vi "Weather Station UI_EX.vi"() -> ()   [LabVIEW 2021]
doc: "This is the main VI in the Weather Station project. It contains the user interface for a temperature warning system. Temperature is retrieved every half second; data is logged when a warning has occurred."
uses:
  WeatherData.ctl
  Instance           2 26Saved   Weather Station UI .vi
panel:
  out "Warning":string
  in  "Lower Limit":dbl=20.0
  in  "Upper Limit":dbl=30.0
  in  "Stop Button":bool
  out "Temperature History":dbl(graph)
  # "Temperature Ranges (C)"
  # "Freeze"
  # "Heat \nStroke"
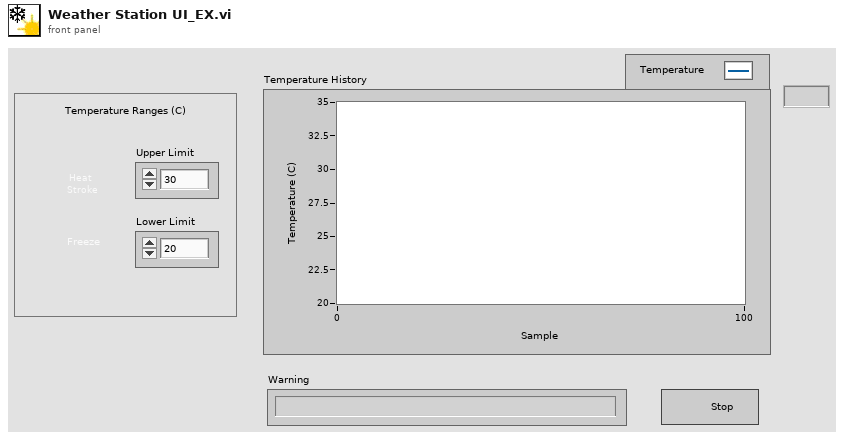
[diagram p1: front panel]
types:
  T1 = enum16{"Acquisition", "Analysis", "Data Log", "Time Check"}
  T2 = typedef "WeatherData.ctl" = cluster{"Current Temperature":dbl, "Max Temperature":dbl, "Min Temperature":dbl, "Warning?":bool, "Warning Text":string}
  T3 = enum16{"open", "replace", "create", "open or create", "replace or create", "replace or create with confirmation"}
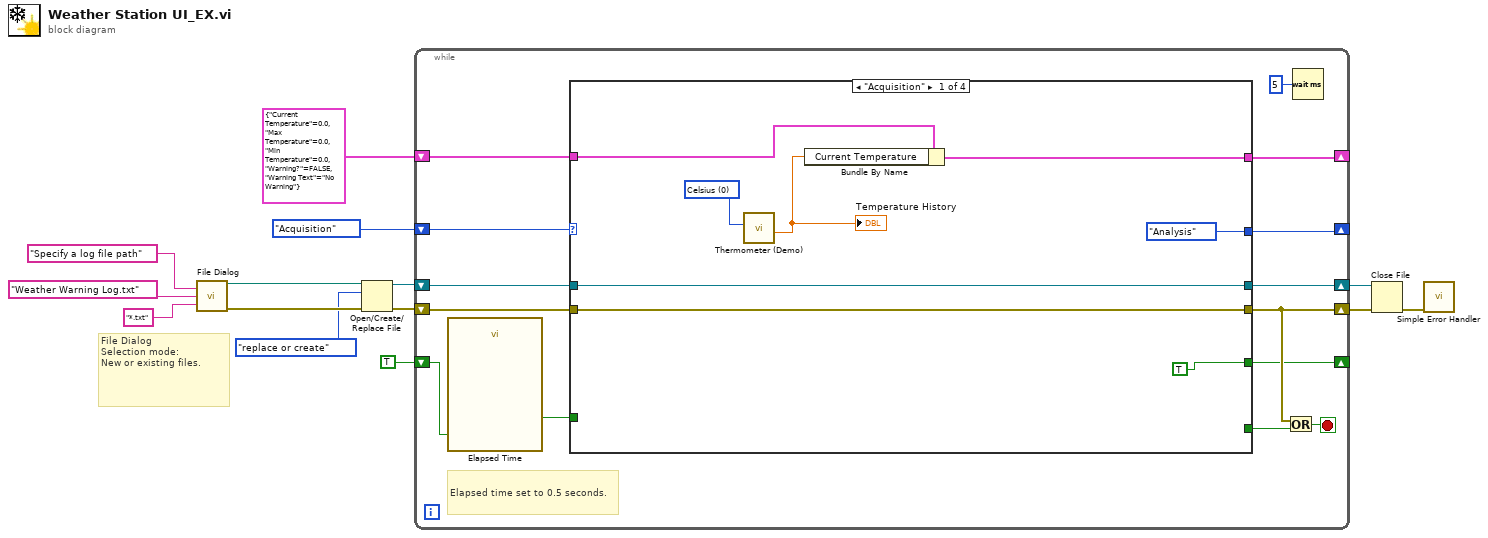
[diagram p0: block diagram]
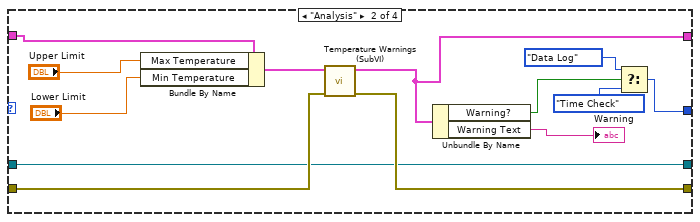
[diagram p2: hidden frame]
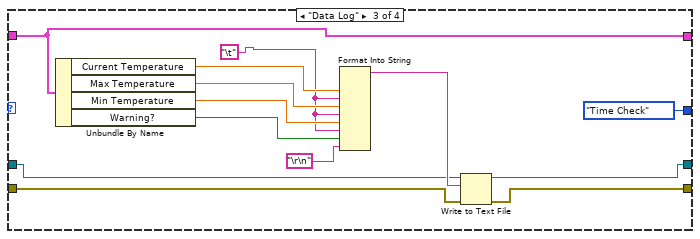
[diagram p3: hidden frame]
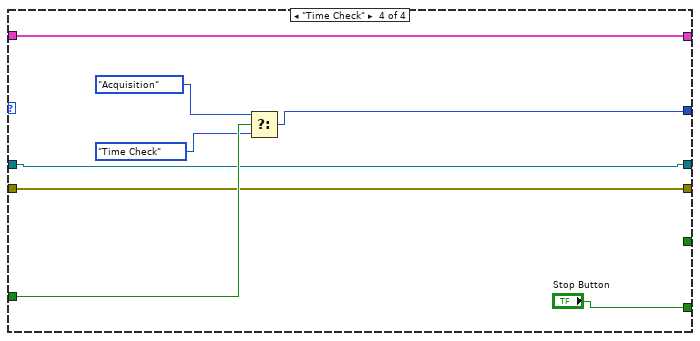
[diagram p4: hidden frame]
diagram:
  # "File Dialog\nSelection mode:\nNew or existing files."
  n1 = call "File Dialog"("prompt"="Specify a log file path", "default name"="Weather Warning Log.txt", "pattern (all files)"="*.txt" ("pattern label")) -> ("selected path"=w8:path, "error out"=w5:errorcluster)  [unwired: 9 in, 2 out]
  n2 = Open/Create/Replace File(file path (use dialog)=w8, error in=w5, operation (0:open)=T3."replace or create") -> (refnum out=w10:refnum<file>, error out=w9:errorcluster)  [unwired: 3 in, 1 out]
  n3 = while {
    shift-right: [w21] -> w14
    shift-left: w9 -> [w28]
    shift-right: [w26] -> w13
    shift-left: w10 -> [w25]
    shift-right: [w16] -> _
    shift-left: TRUE ("stop") -> [w23]
    shift-right: [w17] -> _
    shift-left: T1."Acquisition" ("Enum") -> [w20]
    shift-right: [w18] -> _
    shift-left: T2 {"Current Temperature"=0.0, "Max Temperature"=0.0, "Min Temperature"=0.0, "Warning?"=FALSE, "Warning Text"="No Warning"} ("Weather Data") -> [w19]
    stop <- w27 stop-if-true
    # "Elapsed time set to 0.5 seconds."
    n4 = call "Elapsed Time"("Reset"=w23) -> ("Time has Elapsed"=w22:bool)  [unwired: 11 in, 7 out]
    n5 = case shown="\"Acquisition\"" w20 {
      tunnel: [w35 w44 w51 w64] -> w21
      tunnel: w28 -> [w35 w45 w53 w64]
      tunnel: [w36 w37 w52 w65] -> w26
      tunnel: w25 -> [w36 w37 w54 w65]
      tunnel: w22 -> [_ _ _ w70]
      tunnel: w19 -> [w33 w49 w56 w66]
      tunnel: [w32 w43 w56 w66] -> w18
      tunnel: [T1."Analysis" ("Enum") w40 T1."Time Check" ("f") w67] -> w17
      tunnel: [TRUE _ _ _] -> w16
      tunnel: [_ _ _ "Stop Button"] -> w15
      frame "Acquisition" {
        w34 = u16 0 items=["Celsius", "Fahrenheit"] ("Units (0: Celsius)")
        n6 = call "Thermometer (Demo).vi"("Units (0: Celsius)"=w34) -> ("Temperature Value"=w29:dbl)  [unwired: 10 in]
        "Temperature History" <- w29
        n7 = Bundle By Name(cluster=w33, "Current Temperature"=w29) -> (w32:T2)
      }
      frame "Analysis" {
        n8 = Bundle By Name(cluster=w49, "Max Temperature"="Upper Limit", "Min Temperature"="Lower Limit") -> (w46:T2)
        n9 = call "Temperature Warnings (SubVI).vi"("error in (no error)"=w45, "Weather Data In"=w46) -> ("error out"=w44:errorcluster, "Weather Data Out"=w43:T2)  [unwired: 8 in]
        n10 = Unbundle By Name(w43) -> ("Warning?"=w41:bool, "Warning Text"=→"Warning":string)
        n11 = Select(t=T1."Data Log" ("Enum"), s=w41, f=T1."Time Check") -> (s? t:f=w40:T1)
      }
      frame "Data Log" {
        w57 = "\t"
        n12 = Unbundle By Name(w56) -> ("Current Temperature"=w62:dbl, "Max Temperature"=w61:dbl, "Min Temperature"=w60:dbl, "Warning?"=w59:bool)
        n13 = Format Into String(w62, w57, w61, w57, w60, w57, w59, "\r\n") -> (resulting string=w55:string)  [unwired: 3 in, 1 out]
        n14 = Write to Text File(file (use dialog)=w54, text=w55, error in=w53) -> (refnum out=w52:refnum<file>, error out=w51:errorcluster)  [unwired: 1 in, 1 out]
      }
      frame "Time Check" {
        n15 = Select(t=T1."Acquisition" ("Enum"), s=w70, f=T1."Time Check" ("Enum")) -> (s? t:f=w67:T1)
      }
    }
    n16 = Or(x=w21, y=w15) -> (x .or. y?=w27:bool)
    n17 = Wait (ms)(milliseconds to wait=u32 5 ("y")) -> ()  [unwired: 1 out]
  }
  n18 = Close File(refnum=w13, error in=w14) -> (error out=w12:errorcluster)  [unwired: 1 out]
  n19 = call <vilib>:"Simple Error Handler.vi"("error in (no error)"=w12) -> ()  [unwired: 4 in, 5 out]
